vi "DecodeMaskedBytes.vi"(8 "error in (no error)":errorcluster, 10 "Mask Bytes":u8[](array[numeric]), 11 "Encoded Data":u8[](array[numeric])) -> (0 "error out":errorcluster, 3 "Decoded Data":u8[](array[numeric]))   [LabVIEW 2013, in "WebSockets.lvlib" / "WebSocket.lvclass"]
doc: "Unmasks incoming data. Data sent to the client does not need to be masked."
uses:
  WebSocket.lvclass
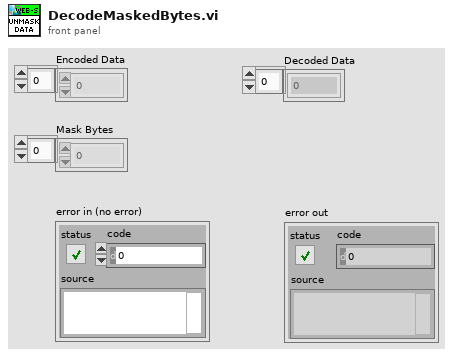
[diagram p1: front panel]
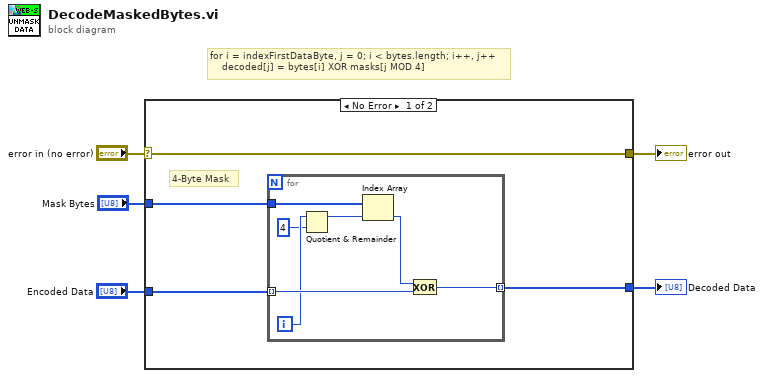
[diagram p0: block diagram]
diagram:
  # "for i = indexFirstDataByte, j = 0; i < bytes.length; i++, j++\n    decoded[j] = bytes[i] XOR masks[j MOD 4]"
  n1 = case shown="No Error" "error in (no error)" {
    selector: "error in (no error)" -> [w9 w17]
    tunnel: "Encoded Data" -> [w8 _]
    tunnel: "Mask Bytes" -> [w7 _]
    tunnel: [w6 _] -> w5
    tunnel: [w9 w17] -> w1
    frame No Error {
      # "4-Byte Mask"
      n2 = for {
        tunnel: w8 -> [w16] mode=indexing
        tunnel: w7 -> [w12]
        tunnel: [w10] -> w6 mode=indexing
        i -> [w15]
        n3 = Quotient & Remainder(x=w15, y=4) -> (x-y*floor(x/y)=w13:i32)  [unwired: 1 out]
        n4 = Index Array(array=w12, index=w13) -> (element=w11:u8)
        n5 = Exclusive Or(1:w16, 2:w11) -> (0:w10:u8)
      }
    }
    frame Error {
    }
  }
  "Decoded Data" <- w5
  "error out" <- w1
